vi "XY Control Panel 3.3.vi"() -> ()   [LabVIEW 2015]
uses:
  states.ctl
  Trash.vi
  Global LED.vi
  Global X.vi
  Global Y.vi
panel:
  out "Units in Trash":dbl
  in  "5822 TEST FAILED\n(INPUT FROM TESTER)":bool
  in  "5822 TEST PASSED\n(INPUT FROM TESTER)":bool
  in  "5822 DETECTED (SENSOR)":bool
  in  "41XX TEST FAILED\n(INPUT FROM TESTER)":bool
  in  "41XX TEST PASSED\n(INPUT FROM TESTER)":bool
  in  "41XX DETECTED (SENSOR)":bool
  in  "INITIAL POSITION":bool
  in  "RESET":bool
  out "SYSTEM WAITING\n FOR INPUT":bool
  out "SYSTEM BUSY":bool
  in  "stop":bool
  out "FAILED":bool
  out "PASSED":bool
  out "SYSTEM STATUS":string
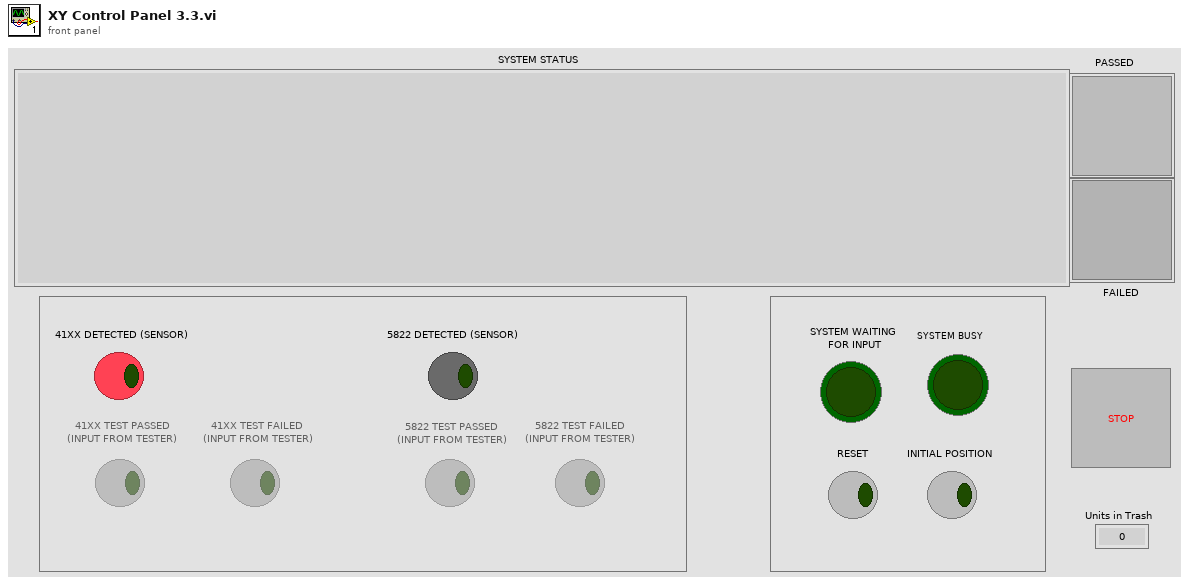
[diagram p1: front panel]
types:
  T1 = typedef "states.ctl" = enum16{"Start", "Initialize", "Idle", "Execute 41XX", "Test 41XX", "Test Passed 41XX", "Test Failed 41XX", "Notify 41XX", "Execute 5822", "Test 5822", "Test Passed 5822", "Test Failed 5822", "Notify 5822", "Reset", "Initial Position"}
  T2 = enum8{"Enabled", "Disabled", "Disabled and Grayed Out"}
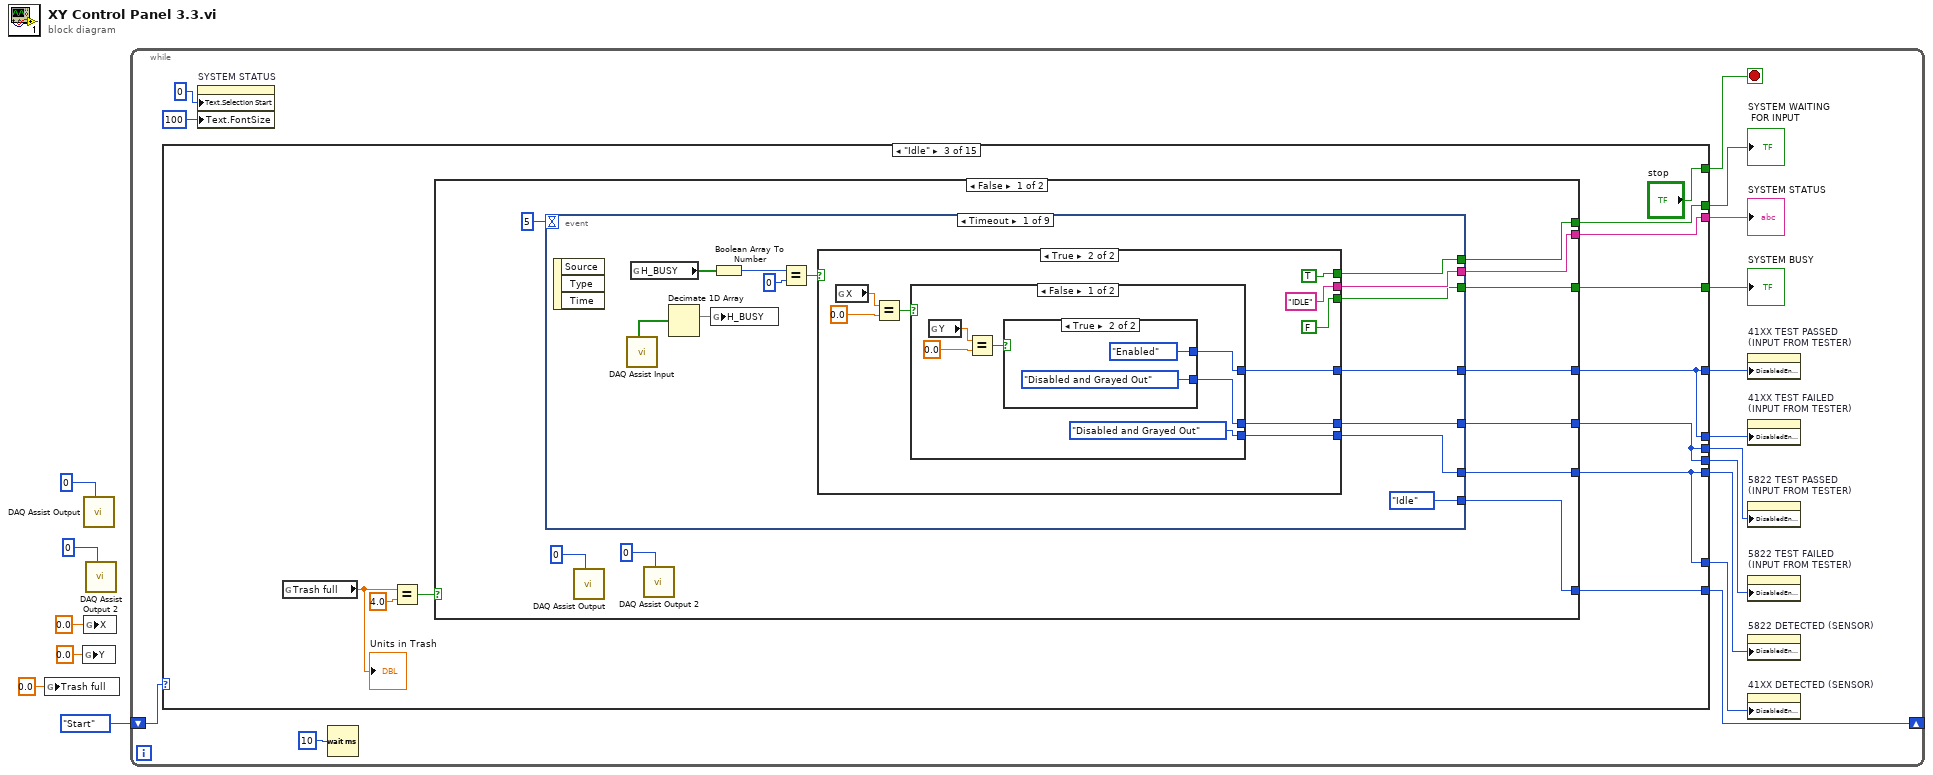
[diagram p0: block diagram]
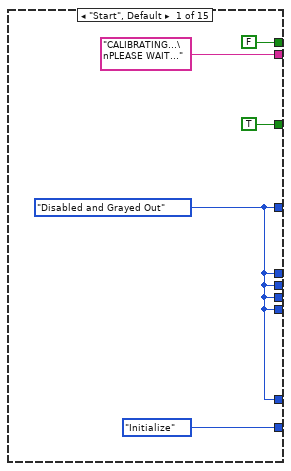
[diagram p2: hidden frame]
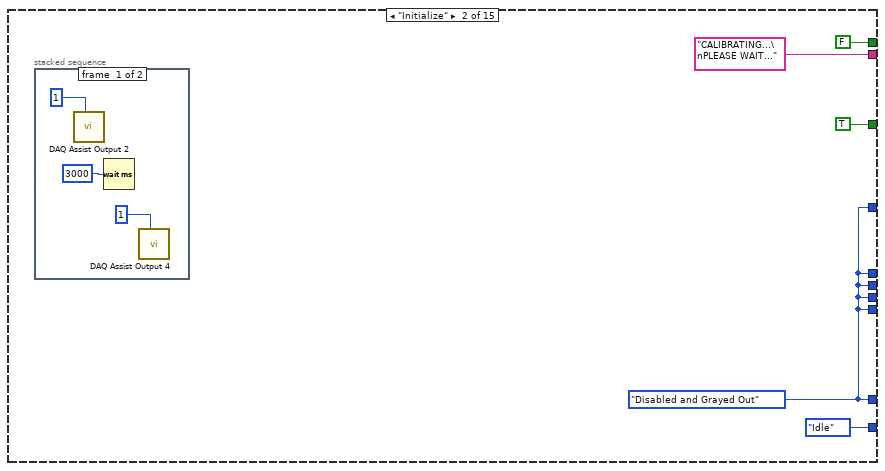
[diagram p3: hidden frame]
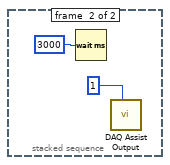
[diagram p4: hidden frame]
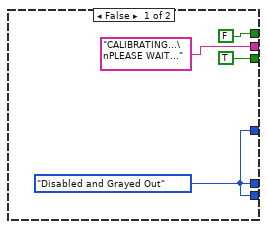
[diagram p5: hidden frame]
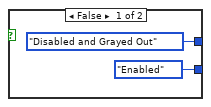
[diagram p6: hidden frame]
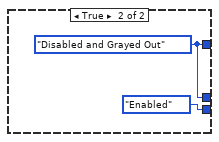
[diagram p7: hidden frame]
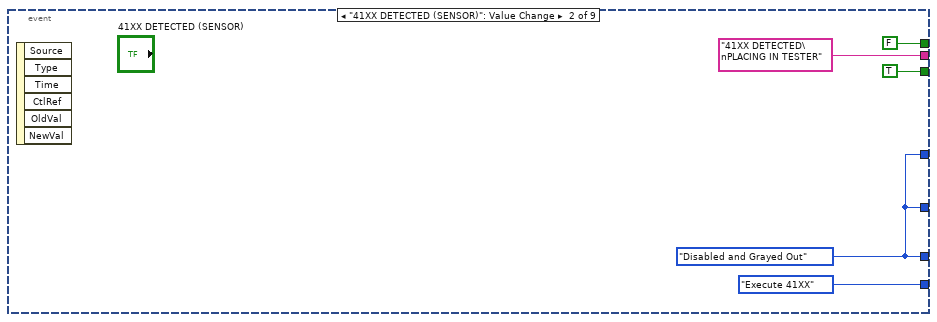
[diagram p8: hidden frame]
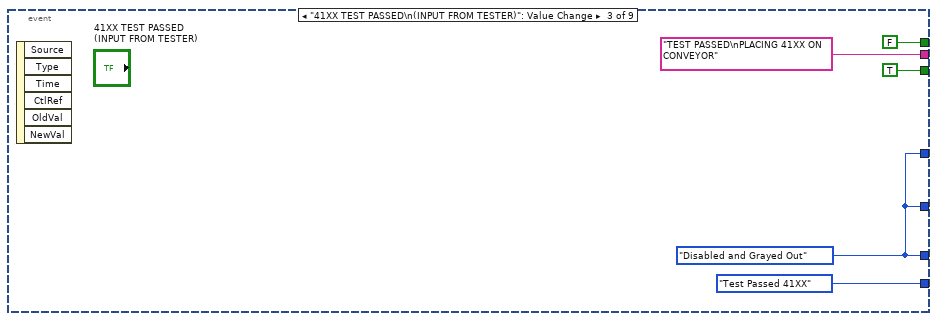
[diagram p9: hidden frame]
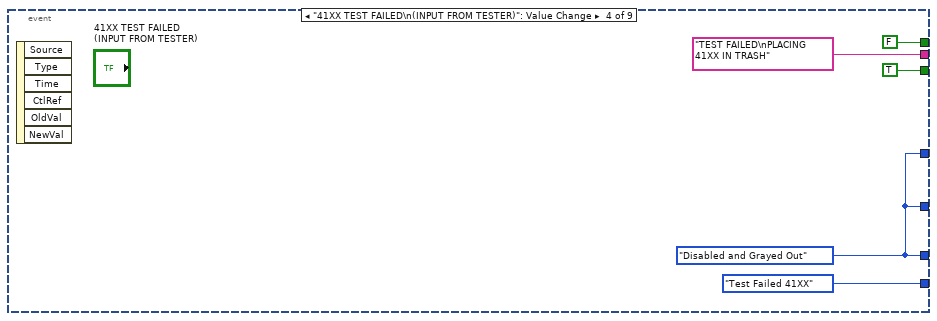
[diagram p10: hidden frame]
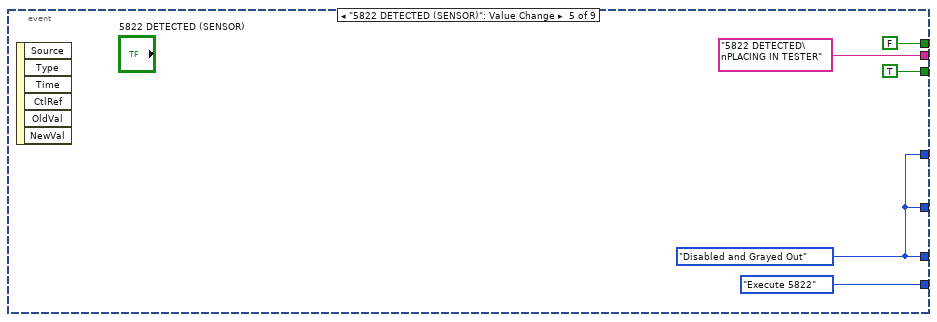
[diagram p11: hidden frame]
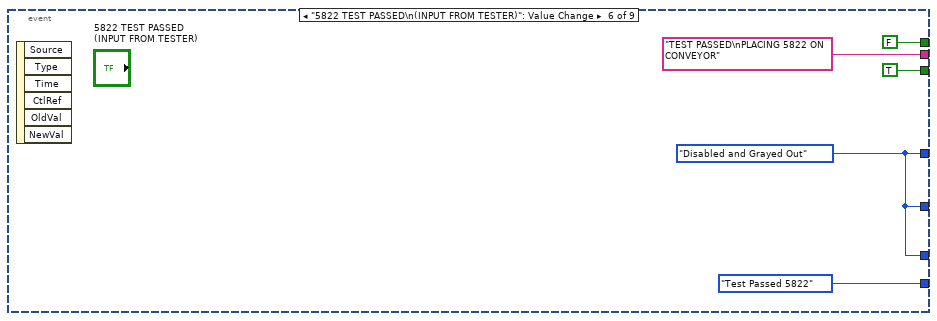
[diagram p12: hidden frame]
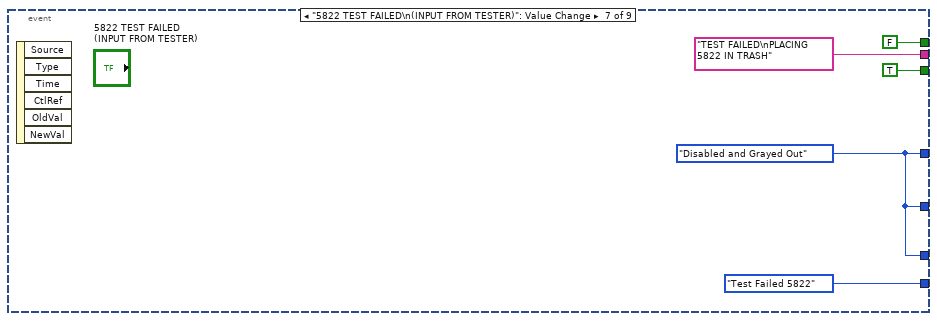
[diagram p13: hidden frame]
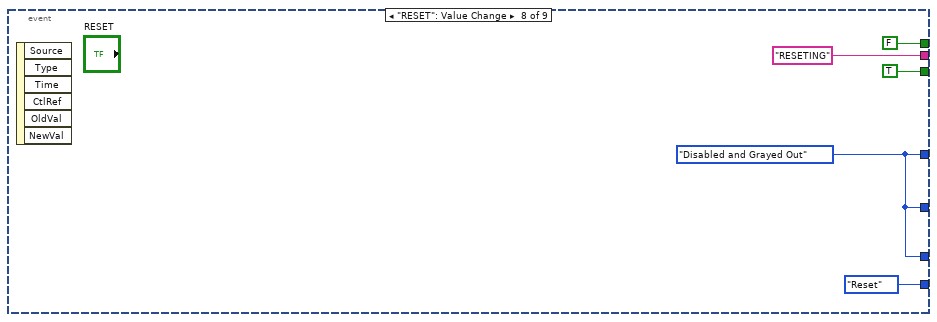
[diagram p14: hidden frame]
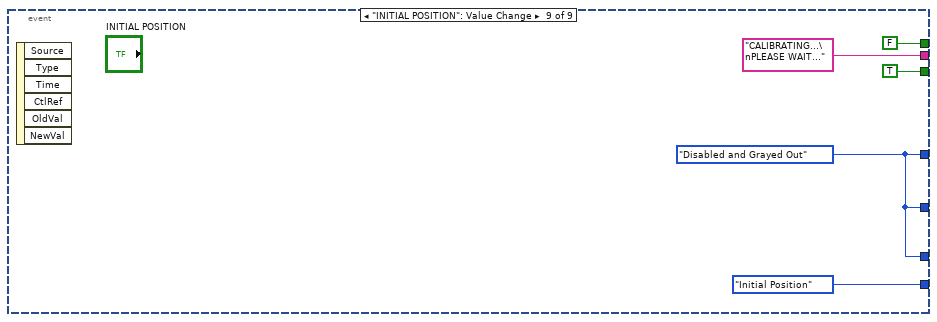
[diagram p15: hidden frame]
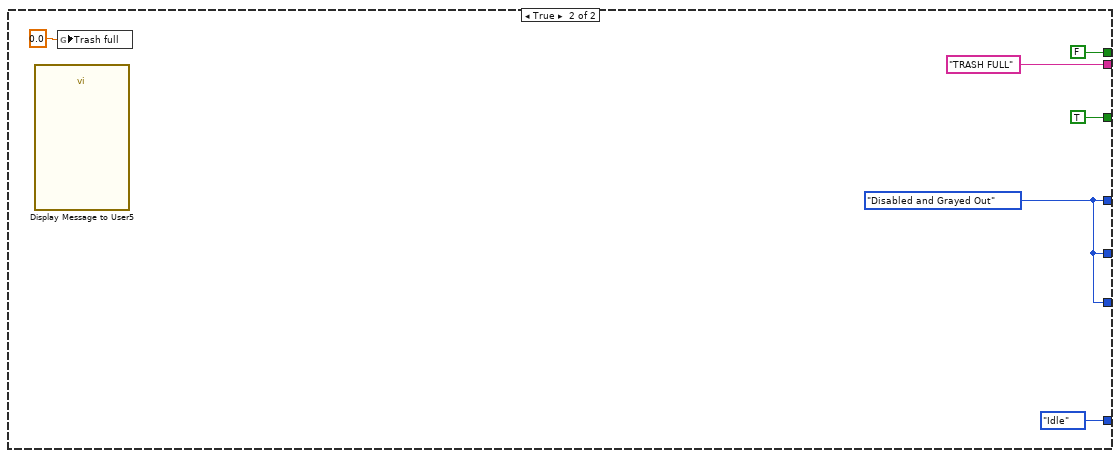
[diagram p16: hidden frame]
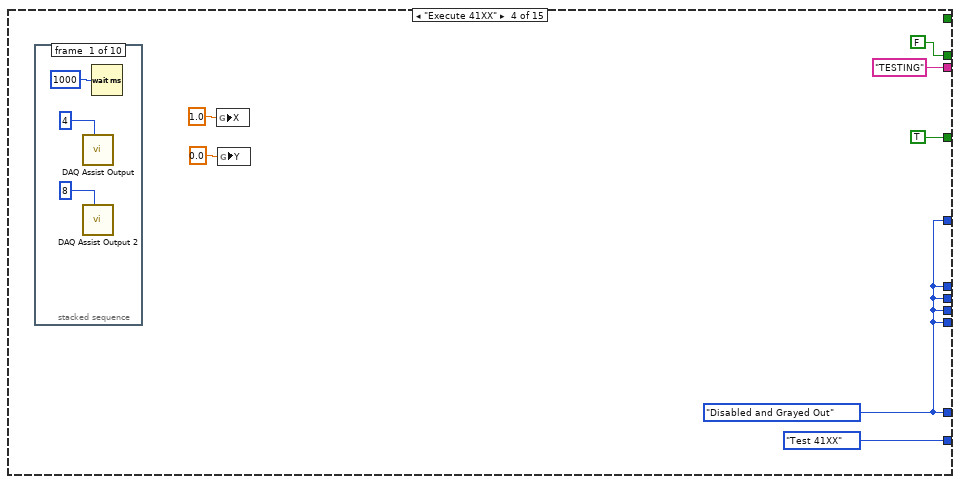
[diagram p17: hidden frame]
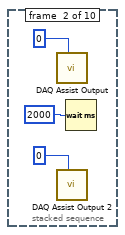
[diagram p18: hidden frame]
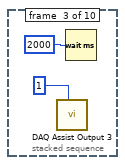
[diagram p19: hidden frame]
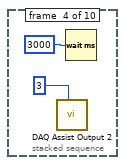
[diagram p20: hidden frame]
diagram:
  n1 = global write "Trash.vi" "Trash full"(0.0 ("Trash full")) -> ()
  n2 = global write "Global Y.vi" "Y"(0.0 ("Y")) -> ()
  n3 = call "DAQ Assist Output.vi"("index"=0) -> ()  [unwired: 11 in]
  n4 = global write "Global X.vi" "X"(0.0 ("X")) -> ()
  n5 = call "DAQ Assist Output 2.vi"("index"=0) -> ()  [unwired: 11 in]
  n6 = while {
    shift-right: [w17] -> _
    shift-left: states."Start" -> [w21]
    stop <- w10 stop-if-true
    n7 = case shown="\"Idle\"" w21 {
      tunnel: [states."Initialize" states."Idle" w46 states."Test 41XX" states."Idle" states."Notify 41XX" states."Notify 41XX" states."Idle" states."Test 5822" states."Idle" states."Notify 5822" states."Notify 5822" states."Idle" states."Idle" states."Idle"] -> w17
      tunnel: ["CALIBRATING...\nPLEASE WAIT..." ("STATUS") "CALIBRATING...\nPLEASE WAIT..." ("STATUS") w45 "TESTING" ("STATUS") "TEST STARTED" ("STATUS") " 41XX TEST PASSED" ("STATUS") "41XX TEST FAILED" ("STATUS") "WAITING FOR CONFIRMATION" ("STATUS") "TESTING" ("STATUS") "TEST STARTED" ("STATUS") "5822 TEST PASSED" ("STATUS") "5822 TEST FAILED" ("STATUS") "WAITING FOR CONFIRMATION" ("STATUS") "RESETING" ("STATUS") "CALIBRATING...\nPLEASE WAIT..." ("STATUS")] -> w16
      tunnel: [w22 w27 w41 w143 w176 w181 w217 w251 w258 w290 w295 w331 w369 w374 w381] -> w15
      tunnel: [w22 w27 w42 w143 w176 w181 w217 w251 w258 w290 w295 w331 w369 w374 w381] -> w14
      tunnel: [w22 w27 w41 w143 w176 w181 w217 w251 w258 w290 w295 w331 w369 w374 w381] -> w13
      tunnel: [FALSE ("INPUT") FALSE ("INPUT") w44 FALSE ("INPUT") TRUE ("INPUT") FALSE ("INPUT") FALSE ("INPUT") TRUE ("INPUT") FALSE ("INPUT") TRUE ("INPUT") FALSE ("INPUT") FALSE ("INPUT") TRUE ("INPUT") FALSE ("INPUT") FALSE ("INPUT")] -> w12
      tunnel: [TRUE ("BUSY") TRUE ("BUSY") w43 TRUE ("BUSY") FALSE ("BUSY") TRUE ("BUSY") TRUE ("BUSY") FALSE ("stop") TRUE ("BUSY") FALSE ("BUSY") TRUE ("BUSY") TRUE ("BUSY") FALSE ("BUSY") TRUE ("BUSY") TRUE ("BUSY")] -> w11
      tunnel: [_ _ "stop" _ _ _ _ _ _ _ _ _ _ _ _] -> w10
      tunnel: [w22 w27 w42 w143 w176 w181 w217 w251 w258 w290 w295 w331 w369 w374 w381] -> w9
      tunnel: [w22 w27 w40 w143 w176 w181 w217 w251 w258 w290 w295 w331 w369 w374 w381] -> w8
      tunnel: [w22 w27 w40 w143 w176 w181 w217 w251 w258 w290 w295 w331 w369 w374 w381] -> w7
      frame "Start", Default {
        w22 = T2."Disabled and Grayed Out" ("Disabled")
      }
      frame "Initialize" {
        w27 = T2."Disabled and Grayed Out" ("Disabled")
        n8 = stacked-sequence {
          frame #0 {
            n9 = call "DAQ Assist Output 2.vi"("index"=1) -> ()  [unwired: 11 in]
            n10 = Wait (ms)(milliseconds to wait=u32 3000) -> ()  [unwired: 1 out]
            n11 = call "DAQ Assist Output 4.vi"("index"=1) -> ()  [unwired: 11 in]
          }
          frame #1 {
            n12 = Wait (ms)(milliseconds to wait=u32 3000) -> ()  [unwired: 1 out]
            n13 = call "DAQ Assist Output.vi"("index"=1) -> ()  [unwired: 11 in]
          }
        }
      }
      frame "Idle" {
        n14 = global read "Trash.vi" "Trash full"() -> (w39:dbl)
        "Units in Trash" <- w39
        n15 = Equal?(x=w39, y=4.0) -> (x = y?=w37:bool)
        n16 = case shown="False" w37 {
          tunnel: [w54 states."Idle"] -> w46
          tunnel: [w53 "TRASH FULL" ("STATUS")] -> w45
          tunnel: [w52 FALSE ("INPUT")] -> w44
          tunnel: [w51 TRUE ("INPUT")] -> w43
          tunnel: [w50 w140] -> w42
          tunnel: [w49 w140] -> w41
          tunnel: [w48 w140] -> w40
          frame False {
            n17 = event shown="[0] Timeout" {
              selector: _ -> [_ _ _ _ _ _ _ _ _]
              dyn-events: _ -> [_ _ _ _ _ _ _ _ _]
              timeout: 5 -> [_ _ _ _ _ _ _ _ _]
              tunnel: [w61 "41XX DETECTED\nPLACING IN TESTER" ("STATUS") "TEST PASSED\nPLACING 41XX ON CONVEYOR" ("STATUS") "TEST FAILED\nPLACING 41XX IN TRASH" ("STATUS") "5822 DETECTED\nPLACING IN TESTER" ("STATUS") "TEST PASSED\nPLACING 5822 ON CONVEYOR" ("STATUS") "TEST FAILED\nPLACING 5822 IN TRASH" ("STATUS") "RESETING" ("STATUS") "CALIBRATING...\nPLEASE WAIT..." ("STATUS")] -> w53
              tunnel: [states."Idle" states."Execute 41XX" states."Test Passed 41XX" states."Test Failed 41XX" states."Execute 5822" states."Test Passed 5822" states."Test Failed 5822" states."Reset" states."Initial Position"] -> w54
              tunnel: [w59 TRUE ("BUSY") TRUE ("BUSY") TRUE ("BUSY") TRUE ("BUSY") TRUE ("BUSY") TRUE ("BUSY") TRUE ("INPUT") TRUE ("INPUT")] -> w51
              tunnel: [w70 w96 w101 w106 w111 w116 w121 w130 w135] -> w50
              tunnel: [w69 w96 w101 w106 w111 w116 w121 w130 w135] -> w49
              tunnel: [w60 FALSE ("INPUT") FALSE ("INPUT") FALSE ("INPUT") FALSE ("INPUT") FALSE ("INPUT") FALSE ("INPUT") FALSE ("INPUT") FALSE ("INPUT")] -> w52
              tunnel: [w67 w96 w101 w106 w111 w116 w121 w130 w135] -> w48
              event Timeout {
                n18 = event-data() -> ()  [unwired: 1 in, 3 out]
                n19 = call "DAQ Assist Input.vi"() -> (7:w66:bool[])  [unwired: 11 in]
                n20 = global read "Global LED.vi" "H_BUSY"() -> (w64:bool[])
                n21 = Decimate 1D Array(w66) -> (w65:bool[])  [unwired: 3 out]
                n22 = global write "Global LED.vi" "H_BUSY"(w65) -> ()
                n23 = Boolean Array To Number(Boolean array=w64) -> (number=w63:u32)
                n24 = Equal?(x=w63, y=u32 0) -> (x = y?=w58:bool)
                n25 = case shown="True" w58 {
                  tunnel: [w74 w83] -> w70
                  tunnel: [w74 w80] -> w69
                  tunnel: [w74 w79] -> w67
                  tunnel: ["CALIBRATING...\nPLEASE WAIT..." ("STATUS") "IDLE" ("STATUS")] -> w61
                  tunnel: [FALSE ("INPUT") TRUE ("INPUT")] -> w60
                  tunnel: [TRUE ("BUSY") FALSE ("BUSY")] -> w59
                  frame False {
                    w74 = T2."Disabled and Grayed Out" ("Disabled")
                  }
                  frame True {
                    n26 = global read "Global X.vi" "X"() -> (w82:dbl)
                    n27 = Equal?(x=w82, y=0.0) -> (x = y?=w78:bool)
                    n28 = case shown="False" w78 {
                      tunnel: [T2."Disabled and Grayed Out" ("Disabled") T2."Enabled" ("Disabled")] -> w83
                      tunnel: [w89 w94] -> w80
                      tunnel: [w84 w94] -> w79
                      frame False {
                        n29 = global read "Global Y.vi" "Y"() -> (w86:dbl)
                        n30 = Equal?(x=w86, y=0.0) -> (x = y?=w85:bool)
                        n31 = case shown="True" w85 {
                          tunnel: [T2."Disabled and Grayed Out" ("Disabled") T2."Enabled" ("Disabled")] -> w89
                          tunnel: [T2."Enabled" ("Disabled") T2."Disabled and Grayed Out" ("Disabled")] -> w84
                          frame False {
                          }
                          frame True {
                          }
                        }
                      }
                      frame True {
                        w94 = T2."Disabled and Grayed Out" ("Disabled")
                      }
                    }
                  }
                }
              }
              event "41XX DETECTED (SENSOR)": Value Change {
                w96 = T2."Disabled and Grayed Out" ("Disabled")
                n32 = event-data() -> ()  [unwired: 1 in, 6 out]
              }
              event "41XX TEST PASSED\n(INPUT FROM TESTER)": Value Change {
                w101 = T2."Disabled and Grayed Out" ("Disabled")
                n33 = event-data() -> ()  [unwired: 1 in, 6 out]
              }
              event "41XX TEST FAILED\n(INPUT FROM TESTER)": Value Change {
                w106 = T2."Disabled and Grayed Out" ("Disabled")
                n34 = event-data() -> ()  [unwired: 1 in, 6 out]
              }
              event "5822 DETECTED (SENSOR)": Value Change {
                w111 = T2."Disabled and Grayed Out" ("Disabled")
                n35 = event-data() -> ()  [unwired: 1 in, 6 out]
              }
              event "5822 TEST PASSED\n(INPUT FROM TESTER)": Value Change {
                w116 = T2."Disabled and Grayed Out" ("Disabled")
                n36 = event-data() -> ()  [unwired: 1 in, 6 out]
              }
              event "5822 TEST FAILED\n(INPUT FROM TESTER)": Value Change {
                w121 = T2."Disabled and Grayed Out" ("Disabled")
                n37 = event-data() -> ()  [unwired: 1 in, 6 out]
              }
              event "RESET": Value Change {
                w130 = T2."Disabled and Grayed Out" ("Disabled")
                n38 = event-data() -> ()  [unwired: 1 in, 6 out]
              }
              event "INITIAL POSITION": Value Change {
                w135 = T2."Disabled and Grayed Out" ("Disabled")
                n39 = event-data() -> ()  [unwired: 1 in, 6 out]
              }
            }
            n40 = call "DAQ Assist Output.vi"("index"=0) -> ()  [unwired: 11 in]
            n41 = call "DAQ Assist Output 2.vi"("index"=0) -> ()  [unwired: 11 in]
          }
          frame True {
            w140 = T2."Disabled and Grayed Out" ("Disabled")
            n42 = call "Display Message to User5"() -> ()  [unwired: 10 in, 2 out]
            n43 = global write "Trash.vi" "Trash full"(0.0 ("Trash full")) -> ()
          }
        }
      }
      frame "Execute 41XX" {
        w143 = T2."Disabled and Grayed Out" ("Disabled")
        n44 = stacked-sequence {
          frame #0 {
            n45 = call "DAQ Assist Output.vi"("index"=4) -> ()  [unwired: 11 in]
            n46 = call "DAQ Assist Output 2.vi"("index"=8) -> ()  [unwired: 11 in]
            n47 = Wait (ms)(milliseconds to wait=u32 1000) -> ()  [unwired: 1 out]
          }
          frame #1 {
            n48 = call "DAQ Assist Output.vi"("index"=0) -> ()  [unwired: 11 in]
            n49 = call "DAQ Assist Output 2.vi"("index"=0) -> ()  [unwired: 11 in]
            n50 = Wait (ms)(milliseconds to wait=u32 2000) -> ()  [unwired: 1 out]
          }
          frame #2 {
            n51 = call "DAQ Assist Output 3.vi"("index"=1) -> ()  [unwired: 11 in]
            n52 = Wait (ms)(milliseconds to wait=u32 2000) -> ()  [unwired: 1 out]
          }
          frame #3 {
            n53 = call "DAQ Assist Output 2.vi"("index"=3) -> ()  [unwired: 11 in]
            n54 = Wait (ms)(milliseconds to wait=u32 3000) -> ()  [unwired: 1 out]
          }
          frame #4 {
            n55 = call "DAQ Assist Output 2.vi"("index"=0) -> ()  [unwired: 11 in]
            n56 = call "DAQ Assist Output.vi"("index"=5) -> ()  [unwired: 11 in]
            n57 = Wait (ms)(milliseconds to wait=u32 3000) -> ()  [unwired: 1 out]
          }
          frame #5 {
            n58 = call "DAQ Assist Output.vi"("index"=0) -> ()  [unwired: 11 in]
            n59 = call "DAQ Assist Output 2.vi"("index"=7) -> ()  [unwired: 11 in]
            n60 = Wait (ms)(milliseconds to wait=u32 2000) -> ()  [unwired: 1 out]
          }
          frame #6 {
            n61 = call "DAQ Assist Output 2.vi"("index"=0) -> ()  [unwired: 11 in]
            n62 = call "DAQ Assist Output 3.vi"("index"=2) -> ()  [unwired: 11 in]
            n63 = Wait (ms)(milliseconds to wait=u32 2000) -> ()  [unwired: 1 out]
          }
          frame #7 {
            n64 = call "DAQ Assist Output 3.vi"("index"=0) -> ()  [unwired: 11 in]
            n65 = call "DAQ Assist Output 2.vi"("index"=3) -> ()  [unwired: 11 in]
            n66 = call "DAQ Assist Output 4.vi"("index"=2) -> ()  [unwired: 11 in]
            n67 = Wait (ms)(milliseconds to wait=u32 2000) -> ()  [unwired: 1 out]
          }
          frame #8 {
            n68 = call "DAQ Assist Output.vi"("index"=3) -> ()  [unwired: 11 in]
            n69 = Wait (ms)(milliseconds to wait=u32 2000) -> ()  [unwired: 1 out]
          }
          frame #9 {
            n70 = call "DAQ Assist Output.vi"("index"=0) -> ()  [unwired: 11 in]
            n71 = call "DAQ Assist Output 2.vi"("index"=0) -> ()  [unwired: 11 in]
          }
        }
        n72 = global write "Global X.vi" "X"(1.0 ("X")) -> ()
        n73 = global write "Global Y.vi" "Y"(0.0 ("Y")) -> ()
      }
      frame "Test 41XX" {
        w176 = T2."Disabled and Grayed Out" ("Disabled")
        n74 = call "Display Message to User"() -> ()  [unwired: 10 in, 2 out]
      }
      frame "Test Passed 41XX" {
        w181 = T2."Disabled and Grayed Out" ("Disabled")
        n75 = stacked-sequence {
          frame #0 {
            n76 = call "DAQ Assist Output 4.vi"("index"=3) -> ()  [unwired: 11 in]
            n77 = call "DAQ Assist Output.vi"("index"=5) -> ()  [unwired: 11 in]
            n78 = Wait (ms)(milliseconds to wait=u32 1000) -> ()  [unwired: 1 out]
            "PASSED" <- TRUE ("PASSED")
          }
          frame #1 {
            n79 = call "DAQ Assist Output 2.vi"("index"=7) -> ()  [unwired: 11 in]
            n80 = call "DAQ Assist Output.vi"("index"=0) -> ()  [unwired: 11 in]
            n81 = Wait (ms)(milliseconds to wait=u32 2000) -> ()  [unwired: 1 out]
          }
          frame #2 {
            n82 = call "DAQ Assist Output 2.vi"("index"=0) -> ()  [unwired: 11 in]
            n83 = call "DAQ Assist Output 3.vi"("index"=1) -> ()  [unwired: 11 in]
            n84 = Wait (ms)(milliseconds to wait=u32 2000) -> ()  [unwired: 1 out]
          }
          frame #3 {
            n85 = call "DAQ Assist Output 2.vi"("index"=3) -> ()  [unwired: 11 in]
            n86 = Wait (ms)(milliseconds to wait=u32 2000) -> ()  [unwired: 1 out]
          }
          frame #4 {
            n87 = call "DAQ Assist Output 2.vi"("index"=0) -> ()  [unwired: 11 in]
            n88 = call "DAQ Assist Output.vi"("index"=6) -> ()  [unwired: 11 in]
            n89 = Wait (ms)(milliseconds to wait=u32 2000) -> ()  [unwired: 1 out]
          }
          frame #5 {
            n90 = call "DAQ Assist Output.vi"("index"=0) -> ()  [unwired: 11 in]
            n91 = call "DAQ Assist Output 2.vi"("index"=9) -> ()  [unwired: 11 in]
            n92 = Wait (ms)(milliseconds to wait=u32 3000) -> ()  [unwired: 1 out]
          }
          frame #6 {
            n93 = call "DAQ Assist Output 3.vi"("index"=2) -> ()  [unwired: 11 in]
            n94 = call "DAQ Assist Output 2.vi"("index"=0) -> ()  [unwired: 11 in]
            n95 = Wait (ms)(milliseconds to wait=u32 2000) -> ()  [unwired: 1 out]
          }
          frame #7 {
            n96 = call "DAQ Assist Output 3.vi"("index"=0) -> ()  [unwired: 11 in]
            n97 = call "DAQ Assist Output 2.vi"("index"=3) -> ()  [unwired: 11 in]
            n98 = Wait (ms)(milliseconds to wait=u32 2000) -> ()  [unwired: 1 out]
          }
          frame #8 {
            n99 = call "DAQ Assist Output.vi"("index"=3) -> ()  [unwired: 11 in]
            n100 = local write "PASSED"(FALSE ("PASSED")) -> ()
            n101 = Wait (ms)(milliseconds to wait=u32 3000) -> ()  [unwired: 1 out]
            n102 = call "DAQ Assist Output 4.vi"("index"=1) -> ()  [unwired: 11 in]
          }
        }
        n103 = global write "Global X.vi" "X"(0.0 ("X")) -> ()
      }
      frame "Test Failed 41XX" {
        w217 = T2."Disabled and Grayed Out" ("Disabled")
        n104 = global read "Trash.vi" "Trash full"() -> (w216:dbl)
        n105 = stacked-sequence {
          frame #0 {
            n106 = call "DAQ Assist Output 4.vi"("index"=4) -> ()  [unwired: 11 in]
            n107 = Wait (ms)(milliseconds to wait=u32 1000) -> ()  [unwired: 1 out]
            n108 = call "DAQ Assist Output.vi"("index"=5) -> ()  [unwired: 11 in]
            "FAILED" <- TRUE ("FAILED")
          }
          frame #1 {
            n109 = call "DAQ Assist Output 2.vi"("index"=7) -> ()  [unwired: 11 in]
            n110 = call "DAQ Assist Output.vi"("index"=0) -> ()  [unwired: 11 in]
            n111 = Wait (ms)(milliseconds to wait=u32 2000) -> ()  [unwired: 1 out]
          }
          frame #2 {
            n112 = call "DAQ Assist Output 2.vi"("index"=0) -> ()  [unwired: 11 in]
            n113 = call "DAQ Assist Output 3.vi"("index"=1) -> ()  [unwired: 11 in]
            n114 = Wait (ms)(milliseconds to wait=u32 2000) -> ()  [unwired: 1 out]
          }
          frame #3 {
            n115 = call "DAQ Assist Output 2.vi"("index"=3) -> ()  [unwired: 11 in]
            n116 = Wait (ms)(milliseconds to wait=u32 2000) -> ()  [unwired: 1 out]
          }
          frame #4 {
            n117 = call "DAQ Assist Output 2.vi"("index"=0) -> ()  [unwired: 11 in]
            n118 = call "DAQ Assist Output.vi"("index"=7) -> ()  [unwired: 11 in]
            n119 = Wait (ms)(milliseconds to wait=u32 2000) -> ()  [unwired: 1 out]
          }
          frame #5 {
            n120 = call "DAQ Assist Output.vi"("index"=0) -> ()  [unwired: 11 in]
            n121 = call "DAQ Assist Output 2.vi"("index"=11) -> ()  [unwired: 11 in]
            n122 = Wait (ms)(milliseconds to wait=u32 3000) -> ()  [unwired: 1 out]
          }
          frame #6 {
            n123 = call "DAQ Assist Output 3.vi"("index"=2) -> ()  [unwired: 11 in]
            n124 = call "DAQ Assist Output 2.vi"("index"=0) -> ()  [unwired: 11 in]
            n125 = Wait (ms)(milliseconds to wait=u32 2000) -> ()  [unwired: 1 out]
          }
          frame #7 {
            n126 = call "DAQ Assist Output 3.vi"("index"=0) -> ()  [unwired: 11 in]
            n127 = call "DAQ Assist Output 2.vi"("index"=3) -> ()  [unwired: 11 in]
            n128 = Wait (ms)(milliseconds to wait=u32 2000) -> ()  [unwired: 1 out]
          }
          frame #8 {
            n129 = call "DAQ Assist Output.vi"("index"=3) -> ()  [unwired: 11 in]
            n130 = local write "FAILED"(FALSE ("FAILED")) -> ()
            n131 = call "DAQ Assist Output 4.vi"("index"=1) -> ()  [unwired: 11 in]
            n132 = Wait (ms)(milliseconds to wait=u32 3000) -> ()  [unwired: 1 out]
          }
        }
        n133 = Increment(x=w216) -> (x+1=w215:dbl)
        n134 = global write "Global X.vi" "X"(0.0 ("X")) -> ()
        n135 = global write "Trash.vi" "Trash full"(w215) -> ()
      }
      frame "Notify 41XX" {
        w251 = T2."Disabled and Grayed Out" ("Disabled")
        n136 = call "Display Message to User2"() -> ()  [unwired: 10 in, 2 out]
      }
      frame "Execute 5822" {
        w258 = T2."Disabled and Grayed Out" ("Disabled")
        n137 = stacked-sequence {
          frame #0 {
            n138 = call "DAQ Assist Output.vi"("index"=3) -> ()  [unwired: 11 in]
            n139 = call "DAQ Assist Output 2.vi"("index"=9) -> ()  [unwired: 11 in]
            n140 = Wait (ms)(milliseconds to wait=u32 1000) -> ()  [unwired: 1 out]
          }
          frame #1 {
            n141 = call "DAQ Assist Output.vi"("index"=0) -> ()  [unwired: 11 in]
            n142 = call "DAQ Assist Output 2.vi"("index"=0) -> ()  [unwired: 11 in]
            n143 = Wait (ms)(milliseconds to wait=u32 2000) -> ()  [unwired: 1 out]
          }
          frame #2 {
            n144 = call "DAQ Assist Output 3.vi"("index"=1) -> ()  [unwired: 11 in]
            n145 = Wait (ms)(milliseconds to wait=u32 2000) -> ()  [unwired: 1 out]
          }
          frame #3 {
            n146 = call "DAQ Assist Output 2.vi"("index"=3) -> ()  [unwired: 11 in]
            n147 = Wait (ms)(milliseconds to wait=u32 3000) -> ()  [unwired: 1 out]
          }
          frame #4 {
            n148 = call "DAQ Assist Output 2.vi"("index"=0) -> ()  [unwired: 11 in]
            n149 = call "DAQ Assist Output.vi"("index"=5) -> ()  [unwired: 11 in]
            n150 = Wait (ms)(milliseconds to wait=u32 3000) -> ()  [unwired: 1 out]
          }
          frame #5 {
            n151 = call "DAQ Assist Output.vi"("index"=0) -> ()  [unwired: 11 in]
            n152 = call "DAQ Assist Output 2.vi"("index"=6) -> ()  [unwired: 11 in]
            n153 = Wait (ms)(milliseconds to wait=u32 2000) -> ()  [unwired: 1 out]
          }
          frame #6 {
            n154 = call "DAQ Assist Output 2.vi"("index"=0) -> ()  [unwired: 11 in]
            n155 = call "DAQ Assist Output 3.vi"("index"=2) -> ()  [unwired: 11 in]
            n156 = Wait (ms)(milliseconds to wait=u32 2000) -> ()  [unwired: 1 out]
          }
          frame #7 {
            n157 = call "DAQ Assist Output 3.vi"("index"=0) -> ()  [unwired: 11 in]
            n158 = call "DAQ Assist Output 2.vi"("index"=3) -> ()  [unwired: 11 in]
            n159 = call "DAQ Assist Output 4.vi"("index"=2) -> ()  [unwired: 11 in]
            n160 = Wait (ms)(milliseconds to wait=u32 2000) -> ()  [unwired: 1 out]
          }
          frame #8 {
            n161 = call "DAQ Assist Output.vi"("index"=3) -> ()  [unwired: 11 in]
            n162 = Wait (ms)(milliseconds to wait=u32 2000) -> ()  [unwired: 1 out]
          }
          frame #9 {
            n163 = call "DAQ Assist Output.vi"("index"=0) -> ()  [unwired: 11 in]
            n164 = call "DAQ Assist Output 2.vi"("index"=0) -> ()  [unwired: 11 in]
          }
        }
        n165 = global write "Global X.vi" "X"(1.0 ("X")) -> ()
        n166 = global write "Global Y.vi" "Y"(1.0 ("Y")) -> ()
      }
      frame "Test 5822" {
        w290 = T2."Disabled and Grayed Out" ("Disabled")
        n167 = call "Display Message to User3"() -> ()  [unwired: 10 in, 2 out]
      }
      frame "Test Passed 5822" {
        w295 = T2."Disabled and Grayed Out" ("Disabled")
        n168 = stacked-sequence {
          frame #0 {
            n169 = call "DAQ Assist Output 4.vi"("index"=3) -> ()  [unwired: 11 in]
            n170 = local write "PASSED"(TRUE ("PASSED")) -> ()
            n171 = call "DAQ Assist Output.vi"("index"=5) -> ()  [unwired: 11 in]
            n172 = Wait (ms)(milliseconds to wait=u32 1000) -> ()  [unwired: 1 out]
          }
          frame #1 {
            n173 = call "DAQ Assist Output 2.vi"("index"=6) -> ()  [unwired: 11 in]
            n174 = call "DAQ Assist Output.vi"("index"=0) -> ()  [unwired: 11 in]
            n175 = Wait (ms)(milliseconds to wait=u32 2000) -> ()  [unwired: 1 out]
          }
          frame #2 {
            n176 = call "DAQ Assist Output 2.vi"("index"=0) -> ()  [unwired: 11 in]
            n177 = call "DAQ Assist Output 3.vi"("index"=1) -> ()  [unwired: 11 in]
            n178 = Wait (ms)(milliseconds to wait=u32 2000) -> ()  [unwired: 1 out]
          }
          frame #3 {
            n179 = call "DAQ Assist Output 2.vi"("index"=3) -> ()  [unwired: 11 in]
            n180 = Wait (ms)(milliseconds to wait=u32 2000) -> ()  [unwired: 1 out]
          }
          frame #4 {
            n181 = call "DAQ Assist Output 2.vi"("index"=0) -> ()  [unwired: 11 in]
            n182 = call "DAQ Assist Output.vi"("index"=6) -> ()  [unwired: 11 in]
            n183 = Wait (ms)(milliseconds to wait=u32 2000) -> ()  [unwired: 1 out]
          }
          frame #5 {
            n184 = call "DAQ Assist Output.vi"("index"=0) -> ()  [unwired: 11 in]
            n185 = call "DAQ Assist Output 2.vi"("index"=9) -> ()  [unwired: 11 in]
            n186 = Wait (ms)(milliseconds to wait=u32 3000) -> ()  [unwired: 1 out]
          }
          frame #6 {
            n187 = call "DAQ Assist Output 3.vi"("index"=2) -> ()  [unwired: 11 in]
            n188 = call "DAQ Assist Output 2.vi"("index"=0) -> ()  [unwired: 11 in]
            n189 = Wait (ms)(milliseconds to wait=u32 2000) -> ()  [unwired: 1 out]
          }
          frame #7 {
            n190 = call "DAQ Assist Output 3.vi"("index"=0) -> ()  [unwired: 11 in]
            n191 = call "DAQ Assist Output 2.vi"("index"=3) -> ()  [unwired: 11 in]
            n192 = Wait (ms)(milliseconds to wait=u32 2000) -> ()  [unwired: 1 out]
          }
          frame #8 {
            n193 = call "DAQ Assist Output.vi"("index"=3) -> ()  [unwired: 11 in]
            n194 = local write "PASSED"(FALSE ("PASSED")) -> ()
            n195 = Wait (ms)(milliseconds to wait=u32 3000) -> ()  [unwired: 1 out]
            n196 = call "DAQ Assist Output 4.vi"("index"=1) -> ()  [unwired: 11 in]
          }
        }
        n197 = global write "Global X.vi" "X"(0.0 ("X")) -> ()
      }
      frame "Test Failed 5822" {
        w331 = T2."Disabled and Grayed Out" ("Disabled")
        n198 = global read "Trash.vi" "Trash full"() -> (w330:dbl)
        n199 = stacked-sequence {
          frame #0 {
            n200 = call "DAQ Assist Output 4.vi"("index"=4) -> ()  [unwired: 11 in]
            n201 = local write "FAILED"(TRUE ("PASSED")) -> ()
            n202 = call "DAQ Assist Output.vi"("index"=5) -> ()  [unwired: 11 in]
            n203 = Wait (ms)(milliseconds to wait=u32 1000) -> ()  [unwired: 1 out]
          }
          frame #1 {
            n204 = call "DAQ Assist Output 2.vi"("index"=6) -> ()  [unwired: 11 in]
            n205 = call "DAQ Assist Output.vi"("index"=0) -> ()  [unwired: 11 in]
            n206 = Wait (ms)(milliseconds to wait=u32 2000) -> ()  [unwired: 1 out]
          }
          frame #2 {
            n207 = call "DAQ Assist Output 2.vi"("index"=0) -> ()  [unwired: 11 in]
            n208 = call "DAQ Assist Output 3.vi"("index"=1) -> ()  [unwired: 11 in]
            n209 = Wait (ms)(milliseconds to wait=u32 2000) -> ()  [unwired: 1 out]
          }
          frame #3 {
            n210 = call "DAQ Assist Output 2.vi"("index"=3) -> ()  [unwired: 11 in]
            n211 = Wait (ms)(milliseconds to wait=u32 2000) -> ()  [unwired: 1 out]
          }
          frame #4 {
            n212 = call "DAQ Assist Output 2.vi"("index"=0) -> ()  [unwired: 11 in]
            n213 = call "DAQ Assist Output.vi"("index"=7) -> ()  [unwired: 11 in]
            n214 = Wait (ms)(milliseconds to wait=u32 2000) -> ()  [unwired: 1 out]
          }
          frame #5 {
            n215 = call "DAQ Assist Output.vi"("index"=0) -> ()  [unwired: 11 in]
            n216 = call "DAQ Assist Output 2.vi"("index"=10) -> ()  [unwired: 11 in]
            n217 = Wait (ms)(milliseconds to wait=u32 3000) -> ()  [unwired: 1 out]
          }
          frame #6 {
            n218 = call "DAQ Assist Output 3.vi"("index"=2) -> ()  [unwired: 11 in]
            n219 = call "DAQ Assist Output 2.vi"("index"=0) -> ()  [unwired: 11 in]
            n220 = Wait (ms)(milliseconds to wait=u32 2000) -> ()  [unwired: 1 out]
          }
          frame #7 {
            n221 = call "DAQ Assist Output 3.vi"("index"=0) -> ()  [unwired: 11 in]
            n222 = call "DAQ Assist Output 2.vi"("index"=3) -> ()  [unwired: 11 in]
            n223 = Wait (ms)(milliseconds to wait=u32 2000) -> ()  [unwired: 1 out]
          }
          frame #8 {
            n224 = call "DAQ Assist Output.vi"("index"=3) -> ()  [unwired: 11 in]
            n225 = local write "FAILED"(FALSE ("PASSED")) -> ()
            n226 = call "DAQ Assist Output 4.vi"("index"=1) -> ()  [unwired: 11 in]
            n227 = Wait (ms)(milliseconds to wait=u32 3000) -> ()  [unwired: 1 out]
          }
        }
        n228 = Increment(x=w330) -> (x+1=w329:dbl)
        n229 = global write "Global X.vi" "X"(0.0 ("X")) -> ()
        n230 = global write "Trash.vi" "Trash full"(w329) -> ()
      }
      frame "Notify 5822" {
        w369 = T2."Disabled and Grayed Out" ("Disabled")
        n231 = call "Display Message to User4"() -> ()  [unwired: 10 in, 2 out]
      }
      frame "Reset" {
        w374 = T2."Disabled and Grayed Out" ("Disabled")
        n232 = call "DAQ Assist Output.vi"("index"=2) -> ()  [unwired: 11 in]
        n233 = call "DAQ Assist Output 2.vi"("index"=2) -> ()  [unwired: 11 in]
      }
      frame "Initial Position" {
        w381 = T2."Disabled and Grayed Out" ("Disabled")
        n234 = flat-sequence {
          frame #0 {
            n235 = Wait (ms)(milliseconds to wait=u32 3000) -> ()  [unwired: 1 out]
            n236 = call "DAQ Assist Output 2.vi"("index"=1) -> ()  [unwired: 11 in]
          }
          frame #1 {
            n237 = Wait (ms)(milliseconds to wait=u32 3000) -> ()  [unwired: 1 out]
            n238 = call "DAQ Assist Output.vi"("index"=1) -> ()  [unwired: 11 in]
          }
        }
      }
    }
    "SYSTEM STATUS" <- w16
    "SYSTEM WAITING\n FOR INPUT" <- w12
    "SYSTEM BUSY" <- w11
    n239 = property on="SYSTEM STATUS" class="Str"("Text.Selection Start"=u32 0 ("Text.Selection:Start"), "Text.FontSize"=u32 100 ("Text.Size:Height")) -> ()  [unwired: 2 in, 2 out]
    n240 = Wait (ms)(milliseconds to wait=u32 10) -> ()  [unwired: 1 out]
    n241 = property on="41XX TEST PASSED\n(INPUT FROM TESTER)" class="Bool"("DisabledEnum"=w15) -> ()  [unwired: 2 in, 2 out]
    n242 = property on="41XX TEST FAILED\n(INPUT FROM TESTER)" class="Bool"("DisabledEnum"=w13) -> ()  [unwired: 2 in, 2 out]
    n243 = property on="5822 TEST PASSED\n(INPUT FROM TESTER)" class="Bool"("DisabledEnum"=w8) -> ()  [unwired: 2 in, 2 out]
    n244 = property on="5822 TEST FAILED\n(INPUT FROM TESTER)" class="Bool"("DisabledEnum"=w7) -> ()  [unwired: 2 in, 2 out]
    n245 = property on="5822 DETECTED (SENSOR)" class="Bool"("DisabledEnum"=w9) -> ()  [unwired: 2 in, 2 out]
    n246 = property on="41XX DETECTED (SENSOR)" class="Bool"("DisabledEnum"=w14) -> ()  [unwired: 2 in, 2 out]
  }
